vi "fgv_local-stop.vi"(7 "cmd":T1) -> (3 "stop":bool)   [LabVIEW 2021]
uses:
  ctrl/ini-stop-read.ctl
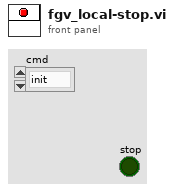
[diagram p1: front panel]
types:
  T1 = typedef "ini-stop-read.ctl" = enum16{"init", "stop", "read"}
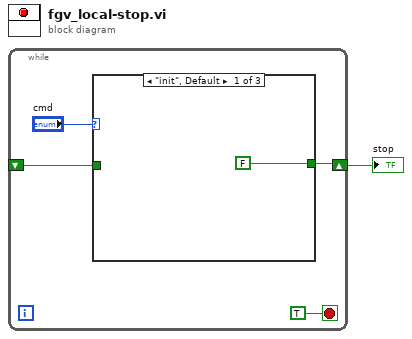
[diagram p0: block diagram]
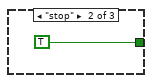
[diagram p2: hidden frame]
diagram:
  n1 = while {
    shift-right: [w3] -> w1
    shift-left: _ -> [w2]
    stop <- TRUE stop-if-true
    n2 = case shown="\"init\", Default" "cmd" {
      tunnel: [FALSE TRUE w8] -> w3
      tunnel: w2 -> [_ _ w8]
      frame "init", Default {
      }
      frame "stop" {
      }
      frame "read" {
      }
    }
  }
  "stop" <- w1
